vi "StartTimer.vi"(1 "exposure time":u32) -> ()   [LabVIEW 2015]
uses:
  ESLSCDLL.dll
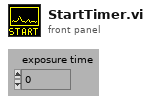
[diagram p1: front panel]
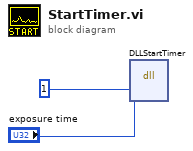
[diagram p0: block diagram]
diagram:
  n1 = dll-call lib="C:/ENTW/PCIE/64bit/lv64/1cam/board.vis/ESLSCDLL.dll" fn="DLLStartTimer"("drv"=u32 1, "exptime"="exposure time") -> ()  [unwired: 6 in, 2 out]
